vi "Select Eye Track Data.vi"(8 "PrevY":u32, 9 "PrevX":u32, 10 "IP Results":T1, 11 "ResetEyeTrack":bool) -> (0 "Xmax":u32, 1 "Ymax":u32, 2 "Xmin":u32, 3 "Ymin":u32)   [LabVIEW 2015]
uses:
  IP Dev Area/IP results.ctl
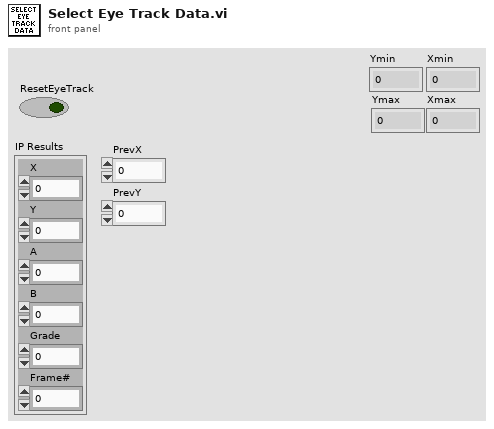
[diagram p1: front panel]
types:
  T1 = typedef "IP results.ctl" = cluster{"X":u16, "Y":u16, "A":dbl, "B":dbl, "Grade":u16, "Frame#":u16}
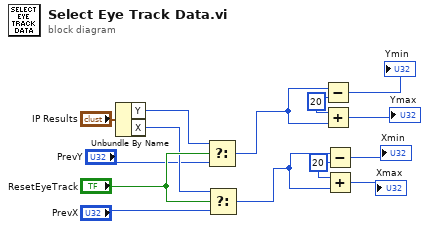
[diagram p0: block diagram]
diagram:
  w9 = u32 20 ("y")
  w8 = u32 20 ("y")
  n1 = Unbundle By Name("IP Results") -> ("Y"=w6:u16, "X"=w4:u16)
  n2 = Select(t=w6, s="ResetEyeTrack", f="PrevY") -> (s? t:f=w5:u32)
  n3 = Select(t=w4, s="ResetEyeTrack", f="PrevX") -> (s? t:f=w3:u32)
  n4 = Subtract(x=w5, y=w8) -> (x-y=→"Ymin":u32)
  n5 = Add(x=w8, y=w5) -> (x+y=→"Ymax":u32)
  n6 = Subtract(x=w3, y=w9) -> (x-y=→"Xmin":u32)
  n7 = Add(x=w9, y=w3) -> (x+y=→"Xmax":u32)
